vi "PH_USB600x_AnalogReader.contents.vi"   [LabVIEW 2014, in "PH_USB600x_AnalogReader.lvlib"]
uses:
  PH_USB600x_AnalogReader.lvlib
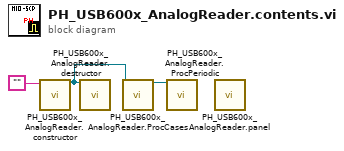
[diagram p0: block diagram]
diagram:
  n1 = call "PH_USB600x_AnalogReader.constructor.vi"("name"="") -> ("i ref out"=w1:refnum<vi>)  [unwired: 16 in, 2 out]
  n2 = call "PH_USB600x_AnalogReader.destructor.vi"("i ref in"=w1) -> ()  [unwired: 18 in, 1 out]
  n3 = call "PH_USB600x_AnalogReader.ProcCases.vi"("i ref in"=w1) -> ("i ref out"=w3:refnum<vi>)  [unwired: 16 in, 2 out]
  n4 = call "PH_USB600x_AnalogReader.ProcPeriodic.vi"("i ref in"=w3) -> ()  [unwired: 16 in, 3 out]
  n5 = call "PH_USB600x_AnalogReader.panel.vi"() -> ()  [unwired: 19 in, 1 out]
